vi "RT Driver VI.vi"(7 "Operation":T1, 11 "Device Reference in":T2 format="%.0x") -> (0 "Error Code":i32)   [LabVIEW 2026, in "Runtime Configuration Support Example Engine.lvlib"]
uses:
  Runtime Configuration Support Example Engine.lvlib
  <vilib>/NI VeriStand/Custom Device API/Custom Device Item Ref.ctl
  <vilib>/NI VeriStand/Custom Device API/Hardware Interface Driver VI Operation.ctl
  <vilib>/NI VeriStand/Custom Device API/Custom Device Channel Type.ctl
  HW Operations.ctl
  Shared/Compiled.Settings.ctl
  <vilib>/NI VeriStand/Custom Device API/Data Access Type.ctl
  Command Loop.vi
  <vilib>/NI VeriStand/Custom Device API/Global Data Refs.vi
  <vilib>/NI VeriStand/Custom Device API/Custom Device API.lvlib
  Shared/Runtime Configuration Support Example Shared.lvlib
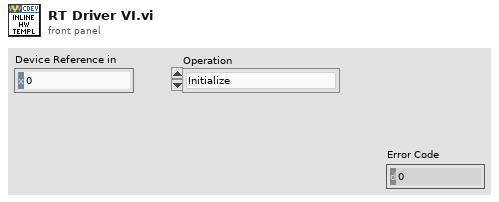
[diagram p1: front panel]
types:
  T1 = typedef "Custom Device API.lvlib/Hardware Interface Driver VI Operation.ctl" = enum16{"Initialize", "Start", "Read Data from HW", "Write Data to HW", "Close"}
  T2 = typedef "Custom Device API.lvlib/Custom Device Item Ref.ctl" = u64
  T3 = typedef "Runtime Configuration Support Example Shared.lvlib/Compiled.Settings.ctl" = cluster{"Name":string, "Inport SignalIDs":i32[], "Outport SignalIDs":i32[], "Inport Channel refs":T2[], "Outport Channel refs":T2[], "Inport Values":dbl[], "Outport Values":dbl[], "Device Error":errorcluster, "Dynamic Config Status":bool, "Response Ref":refnum<queue>}
  T4 = cluster{"Compiled Info":refnum<queue>, "Set HW Val Ref":refnum<queue>, "Get HW Val Ref":refnum<queue>}
  T5 = cluster{"SignalIDs In":i32[], "SignalIDs Out":i32[], "Response Ref":refnum<queue>}
  T6 = cluster{"SignalIDs":i32[], "Values":i32[], "Response Ref":refnum<queue>}
  T7 = typedef "HW Operations.ctl" = enum16{"Initialize", "Set In Val", "Get In Val", "Set Block", "Set Out Val", "Get Out Val", "Get In Array", "Get Out Array"}
  T8 = typedef "Custom Device API.lvlib/Custom Device Channel Type.ctl" = enum16{"Input", "Output"}
  T9 = typedef "Custom Device API.lvlib/Data Access Type.ctl" = enum16{"Read", "Write"}
  T10 = typedef "Custom Device API.lvlib/Data Reference.ctl" = i32
  T11 = cluster{bool, "Inport Values":dbl[], "Outport Values":dbl[], "error IO":errorcluster}
  T12 = cluster{"In Indices":i32[], "Out Indices":i32[], "Response Ref":refnum<queue>}
  T13 = cluster{"Indices":i32[], "Values":i32[], "Response Ref":refnum<queue>}
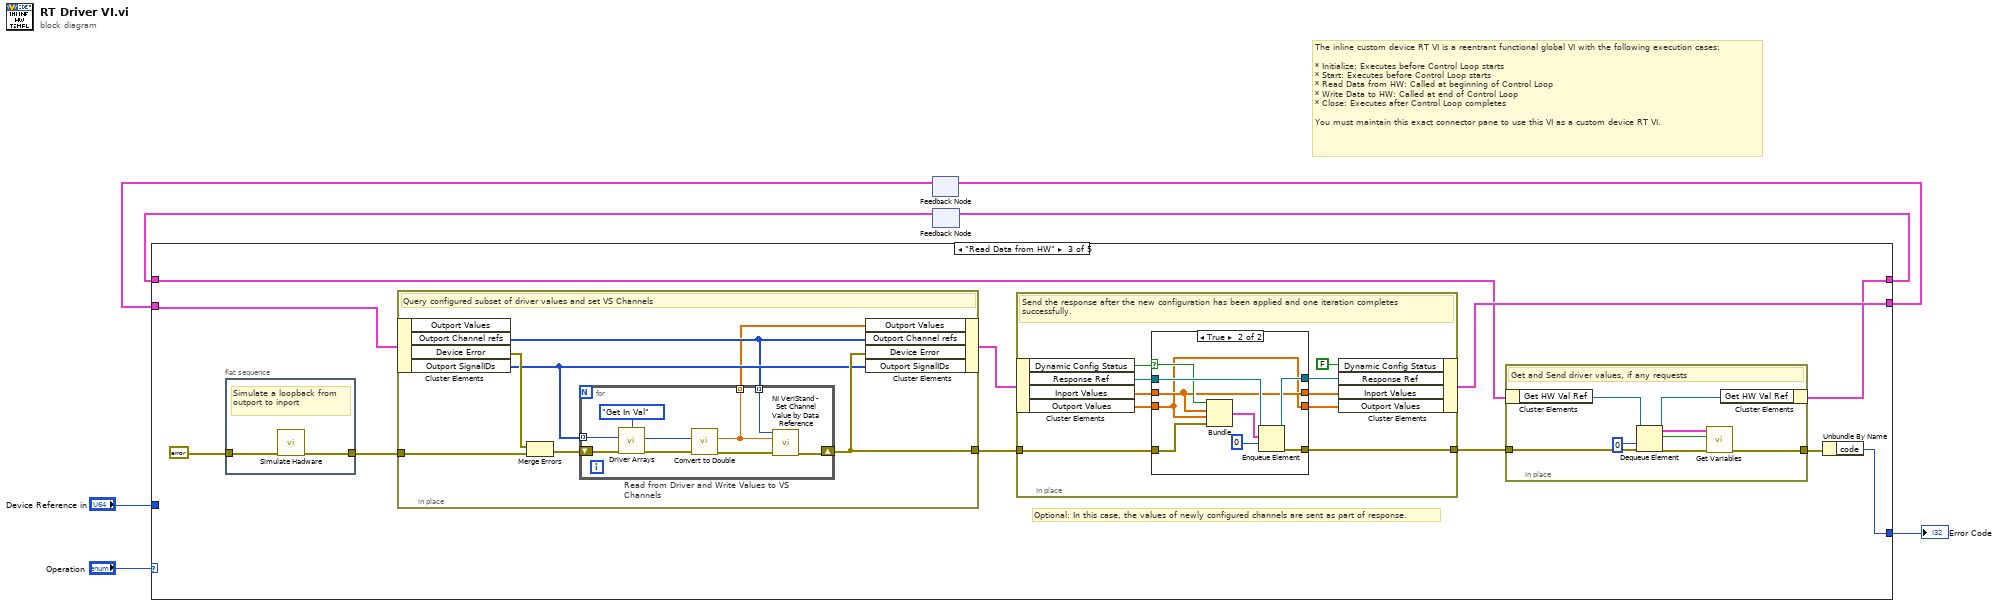
[diagram p0: block diagram]
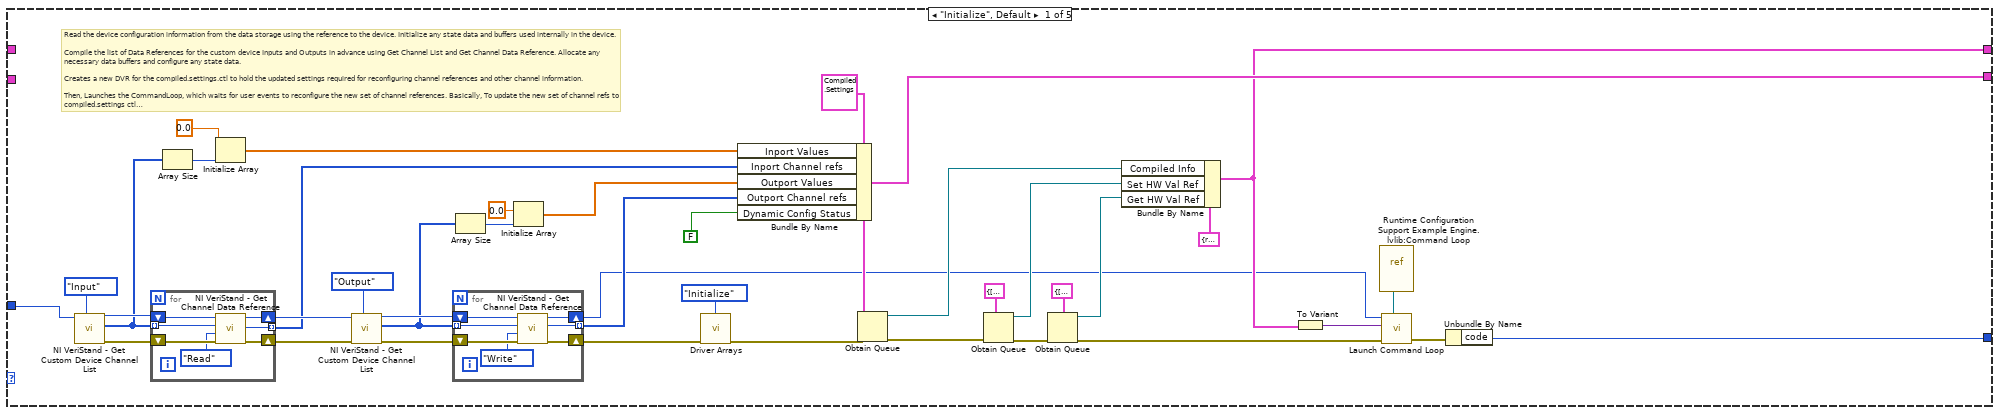
[diagram p2: hidden frame]
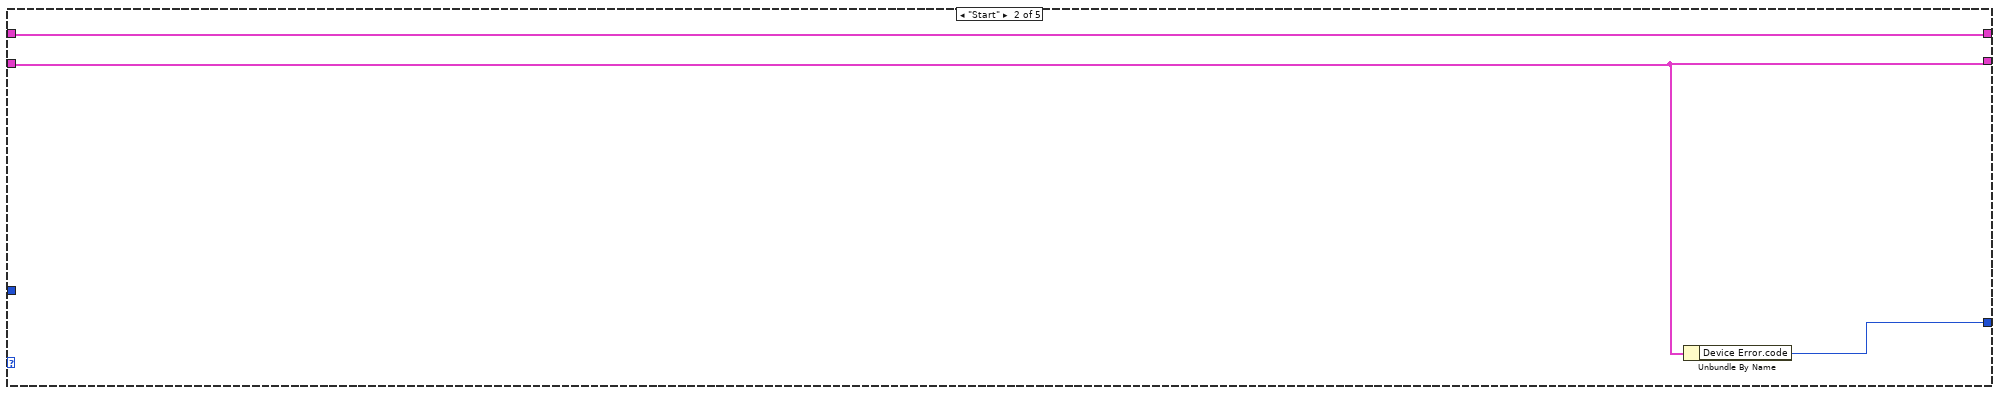
[diagram p3: hidden frame]
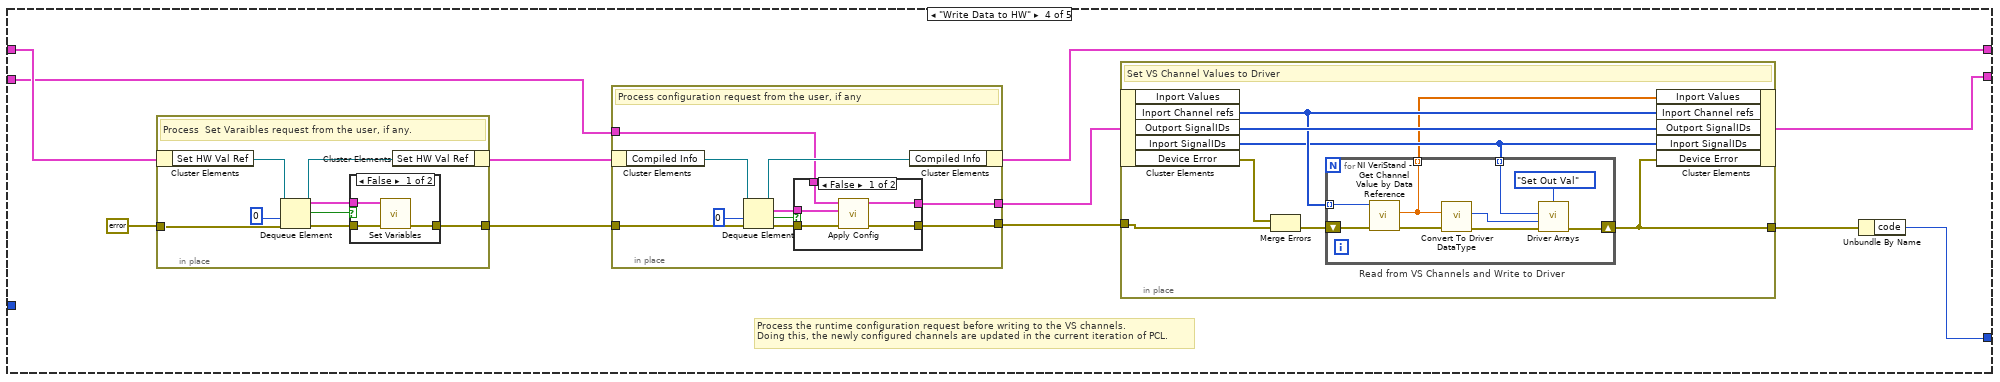
[diagram p5: hidden frame]
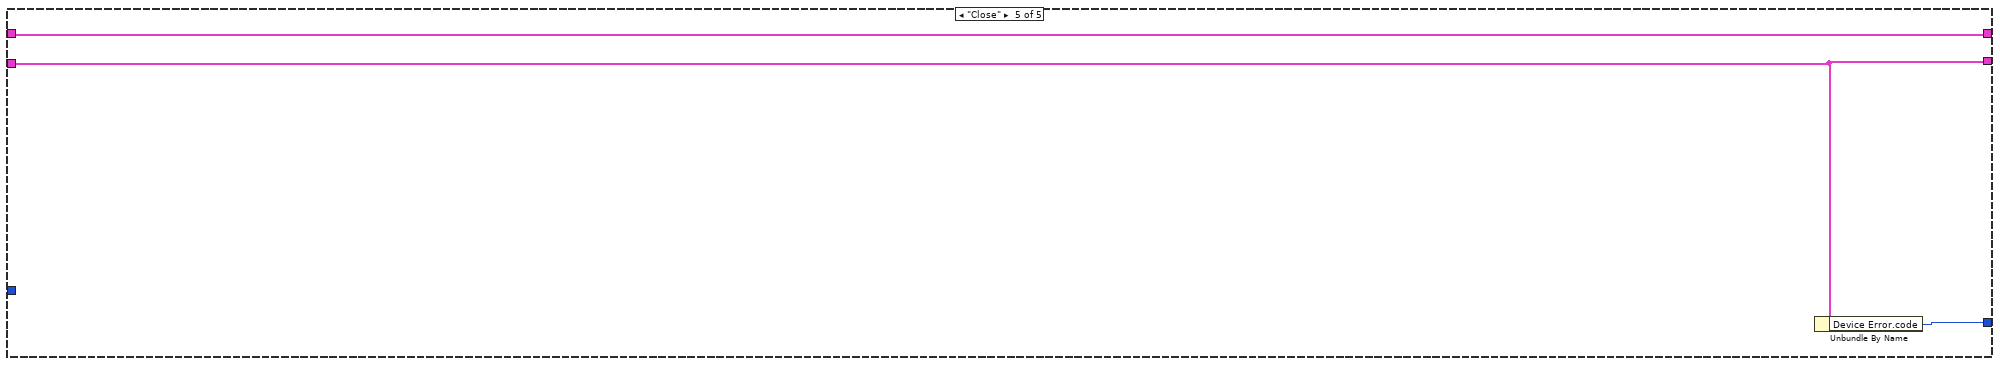
[diagram p8: hidden frame]
diagram:
  # "The inline custom device RT VI is a reentrant functional global VI with the following execution cases:\n\n* Initialize: Executes before Control Loop starts\n* Start: Executes before Control Loop starts\n* Read Data from HW: Called at beginning of Control Loop\n* Write Data to HW: Called at end of Control Loop\n* Close: Executes after Control Loop completes\n\nYou must maintain this exact connector pane to use this VI as a custom device RT VI."
  n1 = feedback #1() -> (w5:T3)  [unwired: 1 out]
  n2 = feedback #2() -> (w1:T4)  [unwired: 1 in]
  n3 = case shown="\"Read Data from HW\"" "Operation" {
    tunnel: [w25 w63 w67 w125 w182] -> w6
    tunnel: w5 -> [_ w63 w69 w128 w182]
    tunnel: "Device Reference in" -> [w11 _ _ _ _]
    tunnel: [w37 w64 w70 w130 w183] -> w3
    tunnel: [w12 w62 w65 w126 w181] -> w2
    tunnel: w1 -> [_ w62 w66 w129 w181]
    frame "Initialize", Default {
      w21 = T3 {"Name"="", "Inport SignalIDs"=[], "Outport SignalIDs"=[], "Inport Channel refs"=[], "Outport Channel refs"=[], "Inport Values"=[], "Outport Values"=[], "Device Error"={"status"=FALSE, "code"=0, "source"=""}, "Dynamic Config Status"=FALSE, "Response Ref"=refnum} ("Compiled.Settings")
      # "Read the device configuration information from the data storage using the reference to the device. Initialize any state data and buffers used internally in the device.\n\nCompile the list of Data References for the custom device Inputs and Outputs in advance using Get Channel List and Get Channel Data Reference. Allocate any necessary data buffers and configure any state data.\n\nCreates a new DVR for the compiled.settings.ctl to hold the updated settings required for reconfiguring channel references and other channel information.\n\nThen, Launches the CommandLoop, which waits for user events to reconfigure the new set of channel references. Basically, To update the new set of channel refs to compiled.settings ctl\n\nYou can't read or write channel values in this case."
      n4 = call <vilib>:"NI VeriStand - Get Custom Device Channel List.vi"("Channel Type"=Custom_Device_Channel_Type."Input", "Device Ref in"=w11) -> ("error out"=w47:errorcluster, "Specified Channel Ref List"=w35:T2[], "Device Ref out"=w36:T2)  [unwired: 1 in, 6 out]
      n5 = for {
        shift-right: [w49] -> w32
        shift-left: w36 -> [w52]
        tunnel: w35 -> [w51] mode=indexing
        shift-right: [w53] -> w45
        shift-left: w47 -> [w54]
        tunnel: [w48] -> w24 mode=indexing
        n6 = call <vilib>:"NI VeriStand - Get Channel Data Reference.vi"("error in (no error)"=w54, "Access"=Data_Access_Type."Read", "Channel Ref in"=w51, "Device Ref in"=w52) -> ("error out"=w53:errorcluster, "Channel Data Reference"=w48:T10, "Device Ref out"=w49:T2)  [unwired: 5 out]
      }
      n7 = Array Size(array=w35) -> (size(s)=w40:i32)
      n8 = Initialize Array(0.0 ("element"), w40) -> (w27:dbl[])
      n9 = call <vilib>:"NI VeriStand - Get Custom Device Channel List.vi"("Channel Type"=Custom_Device_Channel_Type."Output", "error in (no error)"=w45, "Device Ref in"=w32) -> ("error out"=w46:errorcluster, "Specified Channel Ref List"=w29:T2[], "Device Ref out"=w34:T2)  [unwired: 6 out]
      n10 = for {
        tunnel: w29 -> [w58] mode=indexing
        shift-right: [w60] -> w44
        shift-left: w46 -> [w61]
        tunnel: [w56] -> w26 mode=indexing
        shift-right: [w55] -> w10
        shift-left: w34 -> [w59]
        n11 = call <vilib>:"NI VeriStand - Get Channel Data Reference.vi"("error in (no error)"=w61, "Access"=Data_Access_Type."Write", "Channel Ref in"=w58, "Device Ref in"=w59) -> ("error out"=w60:errorcluster, "Channel Data Reference"=w56:T10, "Device Ref out"=w55:T2)  [unwired: 5 out]
      }
      n12 = Array Size(array=w29) -> (size(s)=w30:i32)
      n13 = Initialize Array(0.0 ("element"), w30) -> (w23:dbl[])
      n14 = call "Driver Arrays.vi"("error in"=w44, "Curr Operation"=HW_Operations."Initialize") -> ("error out"=w9:errorcluster)  [unwired: 6 in, 3 out]
      n15 = Bundle By Name(cluster=w21, "Inport Values"=w27, "Inport Channel refs"=w24, "Outport Values"=w23, "Outport Channel refs"=w26, "Dynamic Config Status"=FALSE) -> (w25:T3)
      n16 = Obtain Queue(element data type=w21, error in (no error)=w9) -> (queue out=w15:refnum<queue>, error out=w43:errorcluster)  [unwired: 3 in, 1 out]
      n17 = Obtain Queue(element data type=T6 {"SignalIDs"=[], "Values"=[], "Response Ref"=refnum}, error in (no error)=w43) -> (queue out=w18:refnum<queue>, error out=w42:errorcluster)  [unwired: 3 in, 1 out]
      n18 = Obtain Queue(element data type=T5 {"SignalIDs In"=[], "SignalIDs Out"=[], "Response Ref"=refnum}, error in (no error)=w42) -> (queue out=w17:refnum<queue>, error out=w8:errorcluster)  [unwired: 3 in, 1 out]
      n19 = Bundle By Name(cluster=T4 {"Compiled Info"=refnum, "Set HW Val Ref"=refnum, "Get HW Val Ref"=refnum}, "Compiled Info"=w15, "Set HW Val Ref"=w18, "Get HW Val Ref"=w17) -> (w12:T4)
      n20 = To Variant(anything=w12) -> (Variant=w13:variant)
      n21 = vi-ref "Runtime Configuration Support Example Engine.lvlib:Command Loop.vi"() -> (w14:refnum<vi>)
      n22 = call "Launch Command Loop.vi"("VI Refnum"=w14, "error in"=w8, "Queue Refs"=w13, "Device Reference in"=w10) -> ("error out"=w41:errorcluster)  [unwired: 7 in]
      n23 = Unbundle By Name(w41) -> ("code"=w37:i32)
    }
    frame "Start" {
      n24 = Unbundle By Name(w63) -> ("Device Error.code"=w64:i32)
    }
    frame "Read Data from HW" {
      # "Optional: In this case, the values of newly configured channels are sent as part of response."
      n25 = flat-sequence "Simulate HW" {
        tunnel: [w123] -> w74
        tunnel: errorcluster {"status"=FALSE, "code"=0, "source"=""} ("error in (no error)") -> [w122]
        frame #0 {
          # "Simulate a loopback from outport to inport"
          n26 = call "Simulate Hadware.vi"("error in"=w122) -> ("error out"=w123:errorcluster)  [unwired: 10 in]
        }
      }
      n27 = in-place "In Place Element Structure" {
        in-place-border: w74 -> [w111]
        in-place-border: [w109] -> w71
        # "Query configured subset of driver values and set VS Channels"
        n28 = in-place-cluster #3(w69) -> ("Outport Channel refs"=w107:T2[], "Device Error"=w112:errorcluster, "Outport SignalIDs"=w108:i32[])  [unwired: 1 out]
        n29 = Merge Errors(w112, w111) -> (w110:errorcluster)
        n30 = for "Read from Driver and Write Values to VS Channels" {
          shift-right: [w119] -> w109
          shift-left: w110 -> [w121]
          tunnel: w108 -> [w117] mode=indexing
          tunnel: w107 -> [w114] mode=indexing
          tunnel: [w113] -> w106 mode=indexing
          n31 = call "Driver Arrays.vi"("error in"=w121, "Index"=w117, "Curr Operation"=HW_Operations."Get In Val") -> ("error out"=w120:errorcluster, "Value"=w115:i32)  [unwired: 5 in, 2 out]
          n32 = call "Convert to Double.vi"("error in"=w120, "In"=w115) -> ("error out"=w118:errorcluster, "Out"=w113:dbl)  [unwired: 8 in]
          n33 = call <vilib>:"NI VeriStand - Set Channel Value by Data Reference.vi"("error in (no error)"=w118, "Value"=w113, "Data Reference in"=w114) -> ("error out"=w119:errorcluster)  [unwired: 8 out]
        }
        n34 = in-place-cluster #3("Outport Values"=w106, "Outport Channel refs"=w107, "Device Error"=w109, "Outport SignalIDs"=w108) -> (w68:T3)
      }
      n35 = in-place {
        in-place-border: [w93] -> w73
        in-place-border: w71 -> [w92]
        # "Send the response after the new configuration has been applied and one iteration completes successfully."
        n36 = in-place-cluster #4(w68) -> ("Dynamic Config Status"=w89:bool, "Response Ref"=w91:refnum<queue>, "Inport Values"=w87:dbl[], "Outport Values"=w86:dbl[])
        n37 = case shown="True" w89 {
          selector: w89 -> [_ w100]
          tunnel: [_ w105] -> w93
          tunnel: w91 -> [w96 w103]
          tunnel: [w96 w101] -> w90
          tunnel: w87 -> [w95 w99]
          tunnel: w86 -> [w94 w98]
          tunnel: [w95 w99] -> w85
          tunnel: [w94 w98] -> w84
          tunnel: w92 -> [_ w104]
          frame False {
          }
          frame True {
            n38 = Bundle(w100, "Inport Values"=w99, "Outport Values"=w98, "error IO"=w104) -> (w97:T11)  [unwired: 1 in]
            n39 = Enqueue Element(queue=w103, element=w97, timeout in ms (-1)=0) -> (queue out=w101:refnum<queue>, error out=w105:errorcluster)  [unwired: 1 in, 1 out]
          }
        }
        n40 = in-place-cluster #4("Dynamic Config Status"=FALSE, "Response Ref"=w90, "Inport Values"=w85, "Outport Values"=w84) -> (w67:T3)
      }
      n41 = in-place {
        in-place-border: [w83] -> w72
        in-place-border: w73 -> [w82]
        # "Get and Send driver values, if any requests"
        n42 = in-place-cluster #5(w66) -> ("Get HW Val Ref"=w77:refnum<queue>)
        n43 = Dequeue Element(queue=w77, timeout in ms (-1)=0, error in (no error)=w82) -> (queue out=w79:refnum<queue>, element=w78:T12, timed out?=w80:bool, error out=w81:errorcluster)
        n44 = call "Get Variables.vi"("error in"=w81, "timed out?"=w80, "Data"=w78) -> ("error out"=w83:errorcluster)  [unwired: 8 in]
        n45 = in-place-cluster #5("Get HW Val Ref"=w79) -> (w65:T4)
      }
      n46 = Unbundle By Name(w72) -> ("code"=w70:i32)
    }
    frame "Write Data to HW" {
      # "Process the runtime configuration request before writing to the VS channels.\nDoing this, the newly configured channels are updated in the current iteration of PCL."
      n47 = in-place "In Place Element Structure" {
        in-place-border: [w175] -> w133
        in-place-border: errorcluster {"status"=FALSE, "code"=0, "source"=""} ("error in (no error)") -> [w174]
        # "Process  Set Varaibles request from the user, if any."
        n48 = in-place-cluster #6(w129) -> ("Set HW Val Ref"=w171:refnum<queue>)
        n49 = Dequeue Element(queue=w171, timeout in ms (-1)=0, error in (no error)=w174) -> (queue out=w170:refnum<queue>, element=w173:T13, timed out?=w169:bool, error out=w176:errorcluster)
        n50 = case shown="False" w169 {
          tunnel: w176 -> [w179 w180]
          tunnel: w173 -> [w177 _]
          tunnel: [w178 w180] -> w175
          frame False {
            n51 = call "Set Variables.vi"("error in"=w179, "Data"=w177) -> ("error out"=w178:errorcluster)  [unwired: 9 in]
          }
          frame True {
          }
        }
        n52 = in-place-cluster #6("Set HW Val Ref"=w170) -> (w127:T4)
      }
      n53 = in-place {
        in-place-border: w128 -> [w155]
        in-place-border: [w153] -> w124
        in-place-border: w133 -> [w161]
        in-place-border: [w159] -> w132
        # "Process configuration request from the user, if any"
        n54 = in-place-cluster #7(w127) -> ("Compiled Info"=w157:refnum<queue>)
        n55 = Dequeue Element(queue=w157, timeout in ms (-1)=0, error in (no error)=w161) -> (queue out=w156:refnum<queue>, element=w154:T3, timed out?=w152:bool, error out=w160:errorcluster)
        n56 = case shown="False" w152 {
          tunnel: w160 -> [w166 w168]
          tunnel: [w165 w168] -> w159
          tunnel: w155 -> [w164 w167]
          tunnel: w154 -> [w163 _]
          tunnel: [w162 w167] -> w153
          frame False {
            n57 = call "Apply Config.vi"("error in"=w166, "Data"=w163, "Compiled.Settings in"=w164) -> ("error out"=w165:errorcluster, "Compiled.Settings out"=w162:T3)  [unwired: 7 in]
          }
          frame True {
          }
        }
        n58 = in-place-cluster #7("Compiled Info"=w156) -> (w126:T4)
      }
      n59 = in-place {
        in-place-border: w132 -> [w141]
        in-place-border: [w139] -> w131
        # "Set VS Channel Values to Driver"
        n60 = in-place-cluster #8(w124) -> ("Inport Channel refs"=w137:T2[], "Outport SignalIDs"=w138:i32[], "Inport SignalIDs"=w136:i32[], "Device Error"=w142:errorcluster)  [unwired: 1 out]
        n61 = Merge Errors(w142, w141) -> (w140:errorcluster)
        n62 = for "Read from VS Channels and Write to Driver" {
          shift-right: [w148] -> w139
          shift-left: w140 -> [w151]
          tunnel: w137 -> [w147] mode=indexing
          tunnel: w136 -> [w144] mode=indexing
          tunnel: [w143] -> w135 mode=indexing
          n63 = call <vilib>:"NI VeriStand - Get Channel Value by Data Reference.vi"("error in (no error)"=w151, "Data Reference in"=w147) -> ("error out"=w150:errorcluster, "Value"=w143:dbl)  [unwired: 8 in]
          n64 = call "Convert To Driver DataType.vi"("error in"=w150, "In"=w143) -> ("error out"=w149:errorcluster, "Out"=w145:i32)  [unwired: 8 in]
          n65 = call "Driver Arrays.vi"("error in"=w149, "Value"=w145, "Index"=w144, "Curr Operation"=HW_Operations."Set Out Val") -> ("error out"=w148:errorcluster)  [unwired: 4 in, 3 out]
        }
        n66 = in-place-cluster #8("Inport Values"=w135, "Inport Channel refs"=w137, "Outport SignalIDs"=w138, "Inport SignalIDs"=w136, "Device Error"=w139) -> (w125:T3)
      }
      n67 = Unbundle By Name(w131) -> ("code"=w130:i32)
    }
    frame "Close" {
      n68 = Unbundle By Name(w182) -> ("Device Error.code"=w183:i32)
    }
  }
  "Error Code" <- w3
  n69 = feedback-in #1(w6) -> ()
  n70 = feedback-in #2(w2) -> ()
